vi "getFrameOpenCVIP.vi"(1 "cropY":i32, 2 "cropX":i32, 3 "frameNumber":i32, 4 "Image":T1) -> (0 "return type":i32)   [LabVIEW 2012]
uses:
  <vilib>/vision/Image Controls.llb/IMAQ Image.ctl
  OpenCvGlobals.vi
  <userlib>/OpenCVImProc/CatWalkLabviewDLLd.dll
  <userlib>/OpenCVImProc/CatWalkLabviewDLL.dll
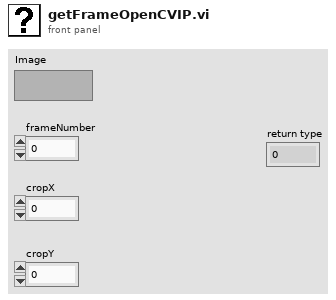
[diagram p1: front panel]
types:
  T1 = typedef "IMAQ Image.ctl" = refnum<image>
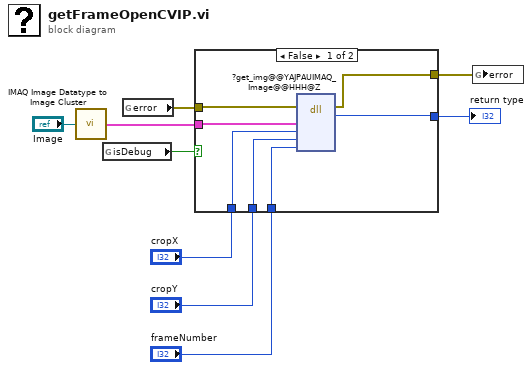
[diagram p0: block diagram]
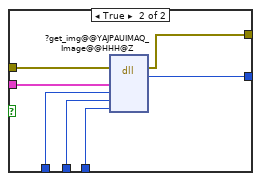
[diagram p2: hidden frame]
diagram:
  n1 = call <vilib>:"IMAQ Image Datatype to Image Cluster.vi"("Image"="Image") -> ("Image (dup)"=w6:cluster{string, u32})
  n2 = global read "OpenCvGlobals.vi" "isDebug"() -> (w9:bool)
  n3 = global read "OpenCvGlobals.vi" "error"() -> (w1:errorcluster)
  n4 = case shown="False" w9 {
    tunnel: [w16 w22] -> w8
    tunnel: [w15 w18] -> w7
    tunnel: w6 -> [w13 w23]
    tunnel: "cropX" -> [w12 w21]
    tunnel: "cropY" -> [w11 w20]
    tunnel: "frameNumber" -> [w10 w19]
    tunnel: w1 -> [w14 w17]
    frame False {
      n5 = dll-call lib="C:/Program Files (x86)/National Instruments/LabVIEW 2012/user.lib/OpenCVImProc/CatWalkLabviewDLL.dll" fn="?get_img@@YAJPAUIMAQ_Image@@HHH@Z"(error in=w14, "image"=w13, "cropX"=w12, "cropY"=w11, "frameNumber"=w10) -> (error out=w15:errorcluster, "return type"=w16:i32)  [unwired: 6 in, 1 out]
    }
    frame True {
      n6 = dll-call lib="C:/Program Files (x86)/National Instruments/LabVIEW 2012/user.lib/OpenCVImProc/CatWalkLabviewDLLd.dll" fn="?get_img@@YAJPAUIMAQ_Image@@HHH@Z"(error in=w17, "image"=w23, "cropX"=w21, "cropY"=w20, "frameNumber"=w19) -> (error out=w18:errorcluster, "return type"=w22:i32)  [unwired: 6 in, 1 out]
    }
  }
  "return type" <- w8
  n7 = global write "OpenCvGlobals.vi" "error"(w7) -> ()
